vi "Load Epics Configuration.vi"(8 "error in (no error)":errorcluster, 11 "Master Configuration in":T1) -> (0 "error out":errorcluster, 3 "Master Configuration out":T1)   [LabVIEW 2014]
uses:
  controls/Master Configuration.ctl
  controls/EPICS Configuration.ctl
  <vilib>/Utility/config.llb/NI_LVConfig.lvlib
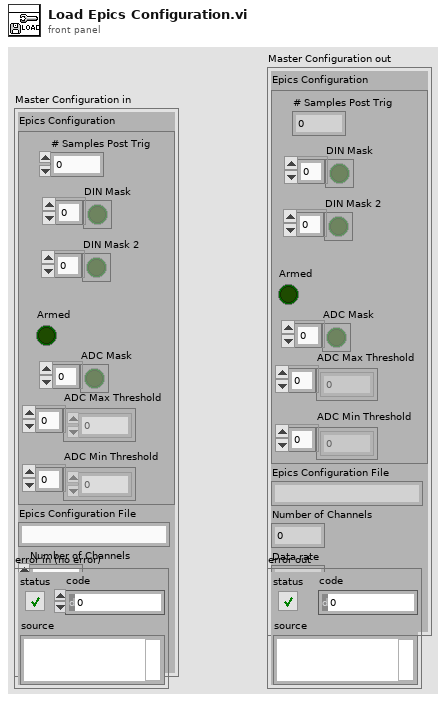
[diagram p1: front panel]
types:
  T1 = typedef "Master Configuration.ctl" = cluster{"Epics Configuration":T2, "Epics Configuration File":string, "Number of Channels":u8, "Data rate":u32, "PM Buffer Size":u32}
  T2 = typedef "EPICS Configuration.ctl" = cluster{"DIN Mask":bool[], "# Samples Post Trig":u32, "Armed":bool, "ADC Mask":bool[], "ADC Max Threshold":dbl[], "ADC Min Threshold":dbl[], "DIN Mask 2":bool[]}
  T3 = typedef "NI_LVConfig.lvlib/Config Data RefNum.ctl" = refnum<k1>
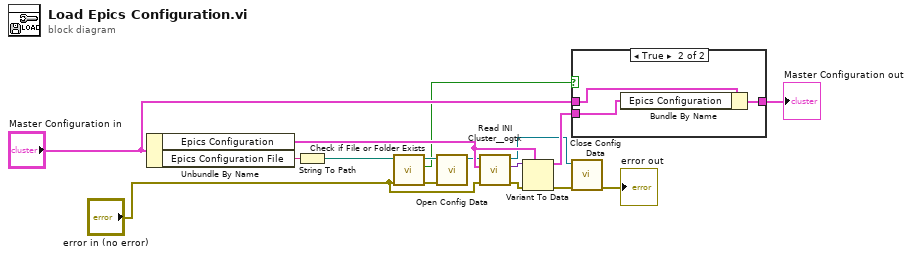
[diagram p0: block diagram]
diagram:
  n1 = Unbundle By Name("Master Configuration in") -> ("Epics Configuration"=w15:T2, "Epics Configuration File"=w7:string)
  n2 = String To Path(string=w7) -> (path=w1:path)
  n3 = call <vilib>:"Check if File or Folder Exists.vi"("error in (no error)"="error in (no error)", "path"=w1) -> ("error out"=w3:errorcluster, "file or folder exists?"=w4:bool, "dup path"=w5:path)  [unwired: 7 in]
  n4 = call <vilib>:"Open Config Data.vi"("error in (no error)"=w3, "configuration file path"=w5) -> ("refnum"=w6:T3)  [unwired: 7 in, 2 out]
  n5 = call <userlib>:"Read INI Cluster__ogtk.vi"("error in (no error)"="error in (no error)", "INI Fomatted Cluster Type"=w15, "refnum"=w6) -> ("error out"=w10:errorcluster, "INI Fomatted Cluster"=w14:variant, "dup refnum"=w9:T3)  [unwired: 4 in, 2 out]
  n6 = Variant To Data(error in=w10, type=w15, Variant=w14) -> (data=w16:T2, error out=w11:errorcluster)
  n7 = case shown="True" w4 {
    tunnel: w16 -> [_ w20]
    tunnel: "Master Configuration in" -> [w17 w19]
    tunnel: [w17 w18] -> w12
    frame False {
    }
    frame True {
      n8 = Bundle By Name(cluster=w19, "Epics Configuration"=w20) -> (w18:T1)
    }
  }
  "Master Configuration out" <- w12
  n9 = call <vilib>:"Close Config Data.vi"("error in (no error)"=w11, "refnum"=w9) -> ("error out"=→"error out":errorcluster)  [unwired: 8 in, 1 out]
